vi "Test Gantry Manifold.vi"() -> ()   [LabVIEW 2011]
uses:
  Gantry Class.lvclass
panel:
  out "error out":errorcluster
  in  "stop":bool
  in  "Array":bool[](array[boolean])=[FALSE, FALSE, FALSE, FALSE, FALSE, FALSE, FALSE, FALSE, FALSE, FALSE, FALSE, FALSE, FALSE, FALSE, FALSE, FALSE]
  in  "Config Folder":path=path "C:/Users/Husker/Desktop/gantry/Config"
  # "line 0"
  # "Each button corresponds\nto a vacuum line on the manifold"
  # "line 1"
  # "line 2"
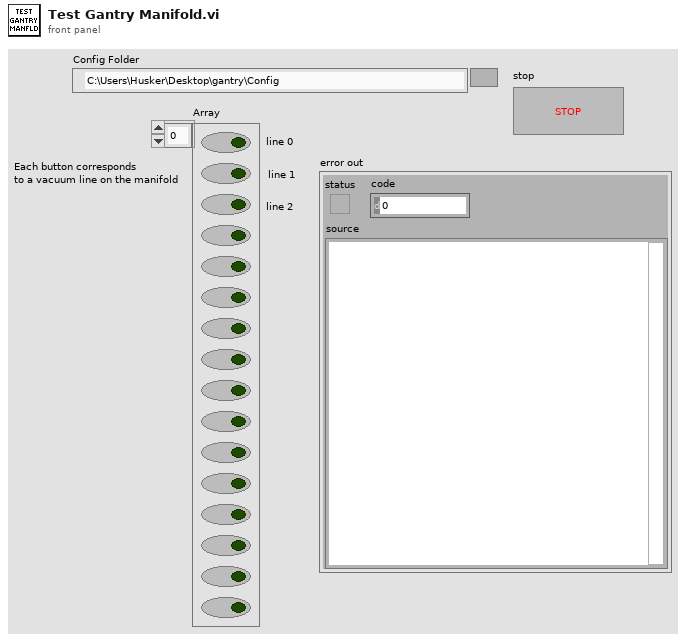
[diagram p1: front panel]
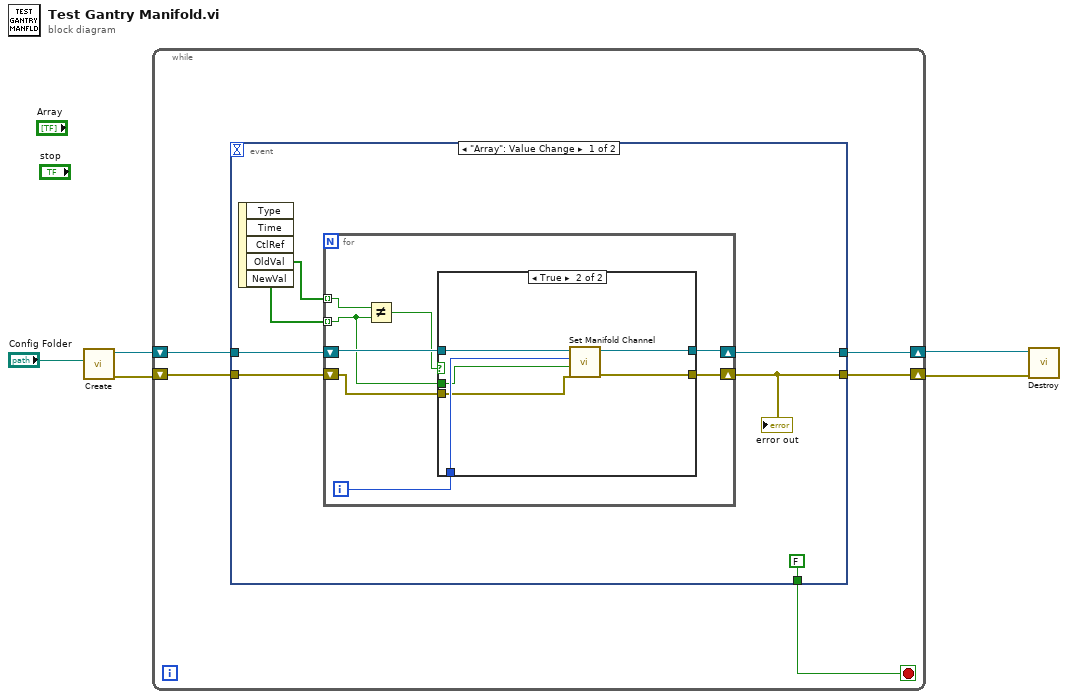
[diagram p0: block diagram]
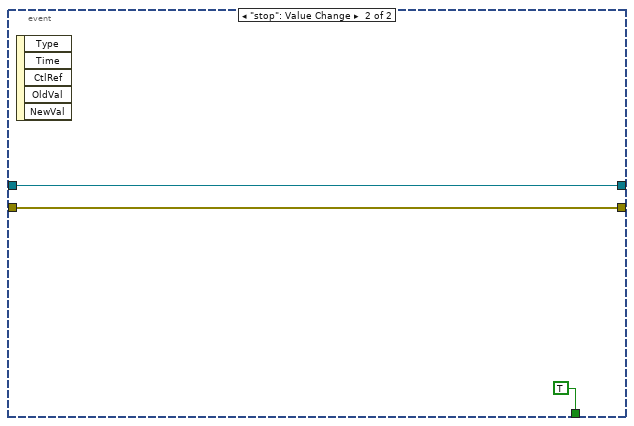
[diagram p3: hidden frame]
diagram:
  n1 = call "Create.vi"("Config Folder"="Config Folder") -> ("error out"=w3:errorcluster, "Gantry Class out"=w4:refnum<class "Gantry Class.lvclass">)  [unwired: 9 in]
  n2 = while {
    shift-right: [w9] -> w2
    shift-left: w4 -> [w10]
    shift-right: [w6] -> w1
    shift-left: w3 -> [w7]
    stop <- w8 stop-if-true
    n3 = event shown="[0] \"Array\": Value Change" {
      selector: _ -> [_ _]
      dyn-events: _ -> [_ _]
      timeout: _ -> [_ _]
      tunnel: w10 -> [w17 w35]
      tunnel: [w16 w35] -> w9
      tunnel: [FALSE TRUE] -> w8
      tunnel: w7 -> [w12 w34]
      tunnel: [w11 w34] -> w6
      event "Array": Value Change {
        n4 = event-data() -> ("OldVal"=w14:bool[], "NewVal"=w13:bool[])  [unwired: 1 in, 3 out]
        n5 = for {
          tunnel: w14 -> [w23] mode=indexing
          tunnel: w13 -> [w20] mode=indexing
          shift-right: [w24] -> w16
          shift-left: w17 -> [w25]
          shift-right: [w18] -> w11
          shift-left: w12 -> [w19]
          i -> [w21]
          n6 = Not Equal?(x=w23, y=w20) -> (x != y?=w22:bool)
          n7 = case shown="True" w22 {
            tunnel: w25 -> [w27 w33]
            tunnel: [w27 w32] -> w24
            tunnel: w21 -> [_ w31]
            tunnel: w20 -> [_ w30]
            tunnel: w19 -> [w26 w29]
            tunnel: [w26 w28] -> w18
            frame False {
            }
            frame True {
              n8 = call "Set Manifold Channel.vi"("error in (no error)"=w29, "On/Off"=w30, "Manifold Channel"=w31, "Gantry Class in"=w33) -> ("error out"=w28:errorcluster, "Gantry Class out"=w32:refnum<class "Gantry Class.lvclass">)  [unwired: 6 in]
            }
          }
        }
        "error out" <- w11
      }
      event "stop": Value Change {
        n9 = event-data() -> ()  [unwired: 1 in, 5 out]
      }
    }
  }
  n10 = call "Destroy.vi"("error in (no error)"=w1, "Gantry Class in"=w2) -> ()  [unwired: 9 in, 1 out]
